vi "Handle Request Timeouts.vi"(10 "Reply Dispatch Loop Data in":T1) -> (2 "Reply Dispatch Loop Data":T1)   [LabVIEW 2020, in "Vecto.lvlib" / "TCPMessaging.lvclass"]
uses:
  TCPMessaging.lvclass
  Reply Dispatch Loop Data.ctl
  Request Registration.ctl
  lv-promises/Promises/Promise/Promise.lvclass
  lv-promises/Promises/Value/Value.lvclass
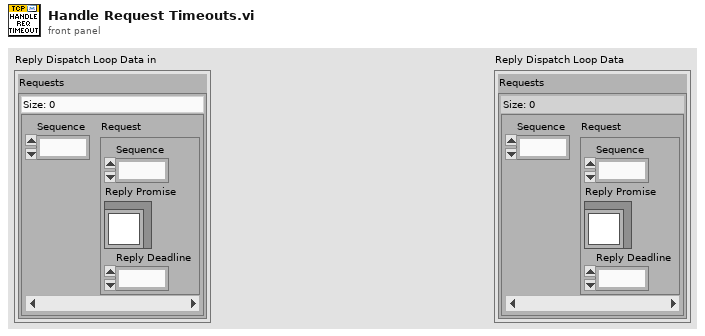
[diagram p1: front panel]
types:
  T1 = typedef "Vecto.lvlib/TCPMessaging.lvclass/Reply Dispatch Loop Data.ctl" = cluster{"Requests":map{u32, T2}}
  T2 = typedef "Vecto.lvlib/TCPMessaging.lvclass/Request Registration.ctl" = cluster{"Sequence":u32, "Reply Promise":refnum<class "Promise.lvclass">, "Reply Deadline":dbl}
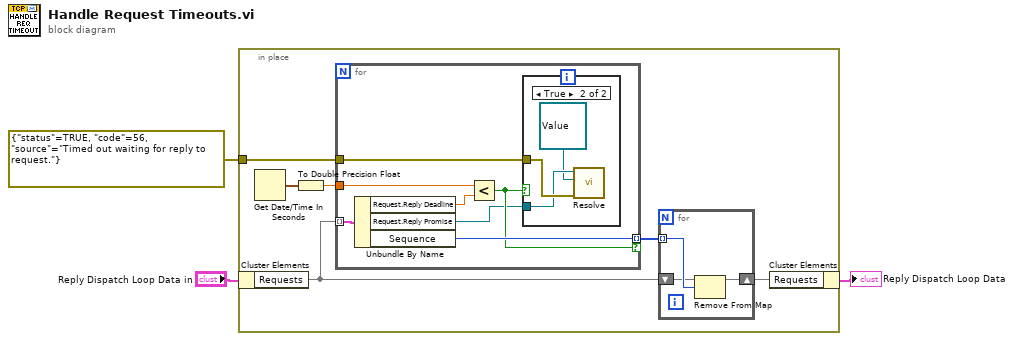
[diagram p0: block diagram]
diagram:
  n1 = in-place {
    in-place-border: errorcluster {"status"=TRUE, "code"=56, "source"="Timed out waiting for reply to request."} ("error constant") -> [w8]
    n2 = in-place-cluster #1("Reply Dispatch Loop Data in") -> ("Requests"=w6:map{u32, T2})
    n3 = Get Date/Time In Seconds() -> (seconds since 1Jan1904=w9:timestamp)
    n4 = To Double Precision Float(number=w9) -> (double precision float=w7:dbl)
    n5 = for {
      tunnel: w8 -> [w13]
      tunnel: w7 -> [w18]
      tunnel: w6 -> [w19] mode=indexing
      tunnel: [w16] -> w4 mode=indexing if=w15
      n6 = Unbundle By Name(w19) -> ("Request.Reply Deadline"=w17:dbl, "Request.Reply Promise"=w14:refnum<class "Promise.lvclass">, "Sequence"=w16:u32)
      n7 = Less?(x=w18, y=w17) -> (x < y?=w15:bool)
      n8 = case shown="True" w15 {
        tunnel: w14 -> [_ w21]
        tunnel: w13 -> [_ w22]
        frame False {
        }
        frame True {
          n9 = call "Resolve.vi"("error in (no error)"=w22, "Result (None)"=refnum<class "Value.lvclass"> refnum ("Result"), "Promise in"=w21) -> ()  [unwired: 7 in, 2 out]
        }
      }
    }
    n10 = for {
      shift-right: [w10] -> w5
      shift-left: w6 -> [w11]
      tunnel: w4 -> [w12] mode=indexing
      n11 = Remove From Map(10:w12, 11:w11) -> (3:w10:map{u32, T2})  [unwired: 2 out]
    }
    n12 = in-place-cluster #1("Requests"=w5) -> (→"Reply Dispatch Loop Data":T1)
  }
